vi "Send Queue data.vi"(7 "Elements in Front":string, 8 "error in (no error)":errorcluster, 9 "message value":variant[](array[variant]), 10 "Elements at Back":string, 11 "CheckPasswordUI in":refnum<class "CheckPasswordUI.lvclass">) -> (0 "error out":errorcluster, 3 "CheckPasswordUI out":refnum<class "CheckPasswordUI.lvclass">)   [LabVIEW 2021, in "CheckPasswordUI.lvclass"]
uses:
  CheckPasswordUI.lvclass
  CheckPasswordUI.lvclass/CheckPasswordUI.ctl
  <userlib>/John_Lib/Queue_Self/Queue_Self.lvlib
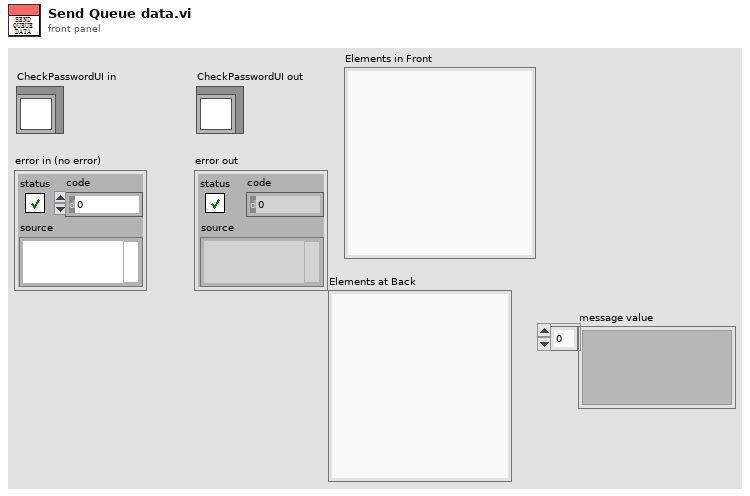
[diagram p1: front panel]
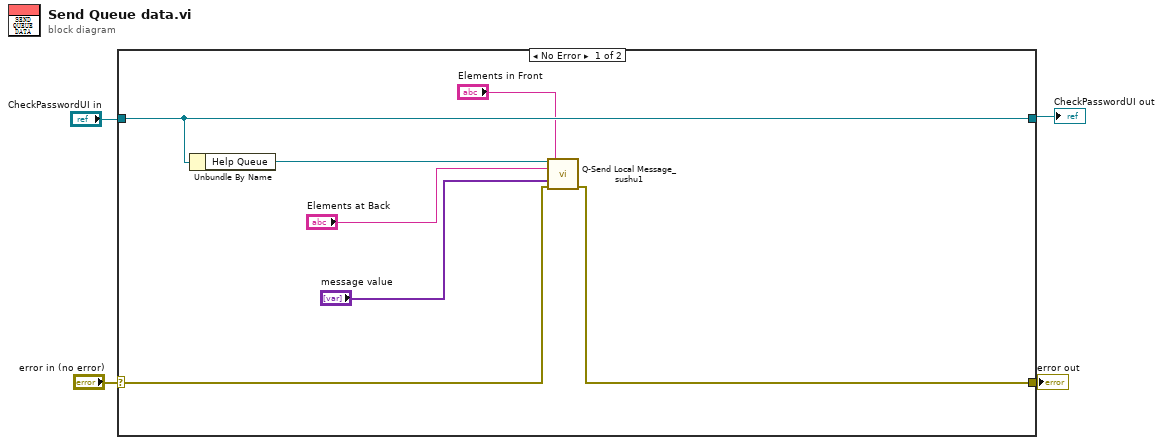
[diagram p0: block diagram]
diagram:
  n1 = case shown="No Error" "error in (no error)" {
    selector: "error in (no error)" -> [w9 w13]
    tunnel: [w8 w13] -> w3
    tunnel: [w11 w12] -> w1
    tunnel: "CheckPasswordUI in" -> [w11 w12]
    frame No Error {
      n2 = Unbundle By Name(w11) -> ("Help Queue"=w10:refnum<queue>)
      n3 = call <userlib>:"Q-Send Local Message_sushu1.vi"("queue in"=w10, "Elements in Front"="Elements in Front", "Elements at Back"="Elements at Back", "message value"="message value", "error in"=w9) -> ("error out"=w8:errorcluster)  [unwired: 8 in, 2 out]
    }
    frame Error {
    }
  }
  "error out" <- w3
  "CheckPasswordUI out" <- w1
